vi "Test Radom with Range.vi"() -> ()   [LabVIEW 2017]
uses:
  9b6d9dd3-ef81-41f5-bf4f-1125acf245ee.vi
panel:
  out "Waveform Chart":dbl(graph)
  out "Random Number":dbl
  in  "B":dbl
  in  "A":dbl=1.0
  in  "stop":bool
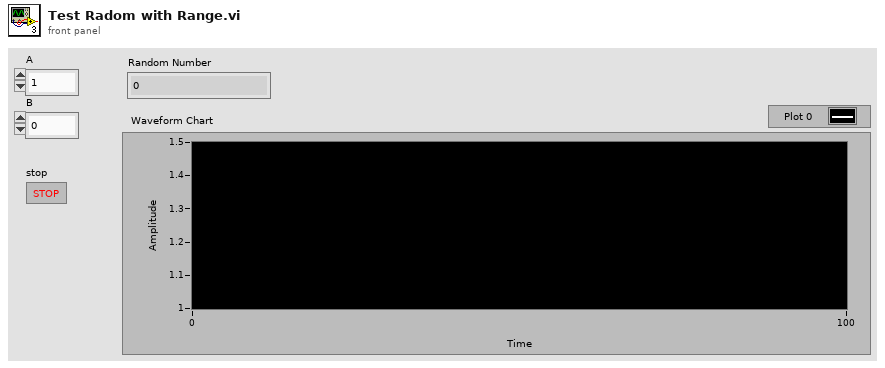
[diagram p1: front panel]
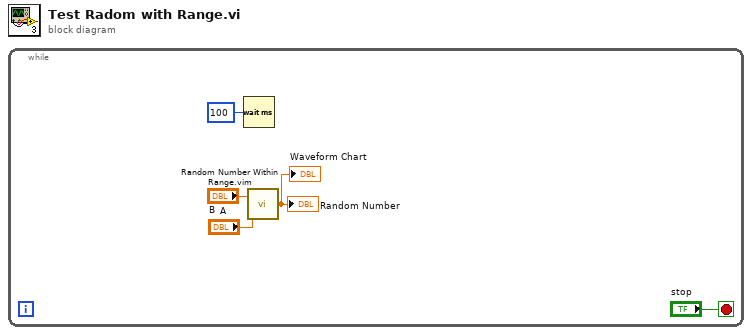
[diagram p0: block diagram]
diagram:
  n1 = while {
    stop <- "stop" stop-if-true
    n2 = Wait (ms)(milliseconds to wait=u32 100) -> ()  [unwired: 1 out]
    n3 = call "Random Number Within Range.vim"("A"="A", "B"="B") -> ("Random Number"=→"Random Number" →"Waveform Chart":dbl)  [unwired: 3 in]
  }
